vi "Start DAQ.vi"(8 "error in (no error)":errorcluster, 10 "Run info in":T1, 11 "Sampling info in":T2={"Channels"=[], "Sampling freq"=0, "Output freq"=0, "Update freq"=0, "Steps per rev"=0, "Counts per rev"=0, "Amplifier"="", "Motor driver"="", "Step bit"=0, "Max speed"=0.0, "Max accel"=0.0, "Pos gain"=0.0, "Vel gain"=0.0, "counter"="Dev1/ctr0"} {"Channels"."Hi cutoff" items=["500"=500.0, "1k"=1000.0, "5k"=5000.0, "10k"=10000.0, "20k"=20000.0]; "Channels"."Lo cutoff" items=["0.1"=0.1, "1"=1.0, "10"=10.0, "100"=100.0, "300"=300.0]; "Channels"."Gain" items=["x100"=100, "x1000"=1000, "x10000"=10000]}) -> (0 "error out":errorcluster, 1 "start time":timestamp, 2 "Run info":T1, 3 "Sampling info out":T2={"Channels"=[], "Sampling freq"=0, "Output freq"=0, "Update freq"=0, "Steps per rev"=0, "Counts per rev"=0, "Amplifier"="", "Motor driver"="", "Step bit"=0, "Max speed"=0.0, "Max accel"=0.0, "Pos gain"=0.0, "Vel gain"=0.0, "counter"="Dev1/ctr0"} {"Channels"."Hi cutoff" items=["500"=500.0, "1k"=1000.0, "5k"=5000.0, "10k"=10000.0, "20k"=20000.0]; "Channels"."Lo cutoff" items=["0.1"=0.1, "1"=1.0, "10"=10.0, "100"=100.0, "300"=300.0]; "Channels"."Gain" items=["x100"=100, "x1000"=1000, "x10000"=10000]})   [LabVIEW 2012]
uses:
  Sampling info.ctl
  Channel.ctl
  Run info.ctl
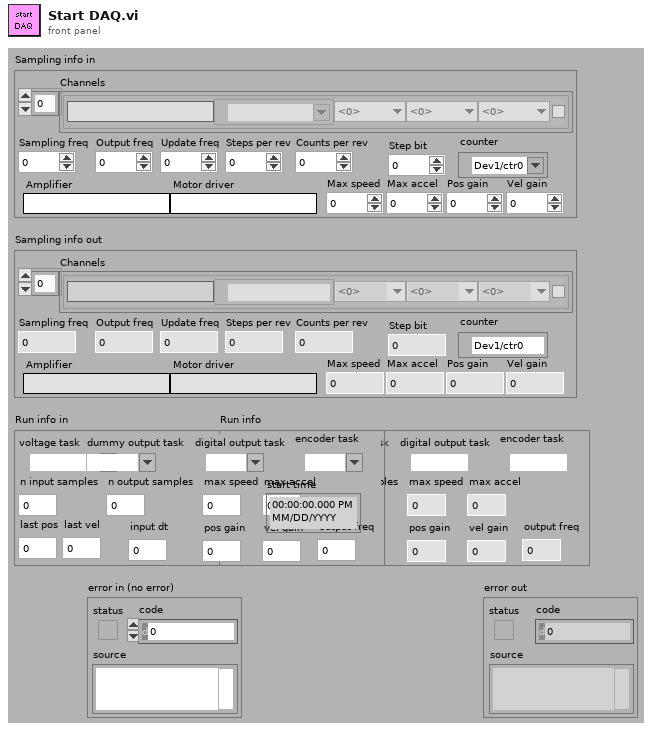
[diagram p1: front panel]
types:
  T1 = typedef "Run info.ctl" = cluster{"voltage task":refnum<k21>, "dummy output task":refnum<k21>, "digital output task":refnum<k21>, "encoder task":refnum<k21>, "n input samples":i32, "n output samples":i32, "max speed":dbl, "max accel":dbl, "last pos":dbl, "last vel":dbl, "pos gain":dbl, "vel gain":dbl, "input dt":dbl, "output freq":dbl}
  T2 = typedef "Sampling info.ctl" = cluster{"Channels":T3[], "Sampling freq":i32, "Output freq":i32, "Update freq":i32, "Steps per rev":i32, "Counts per rev":i32, "Amplifier":string, "Motor driver":string, "Step bit":u8, "Max speed":dbl, "Max accel":dbl, "Pos gain":dbl, "Vel gain":dbl, "counter":tag}
  T3 = typedef "Channel.ctl" = cluster{"Name":string, "Chan":tag, "Gain":u16, "Lo cutoff":dbl, "Hi cutoff":dbl, "Notch":bool}
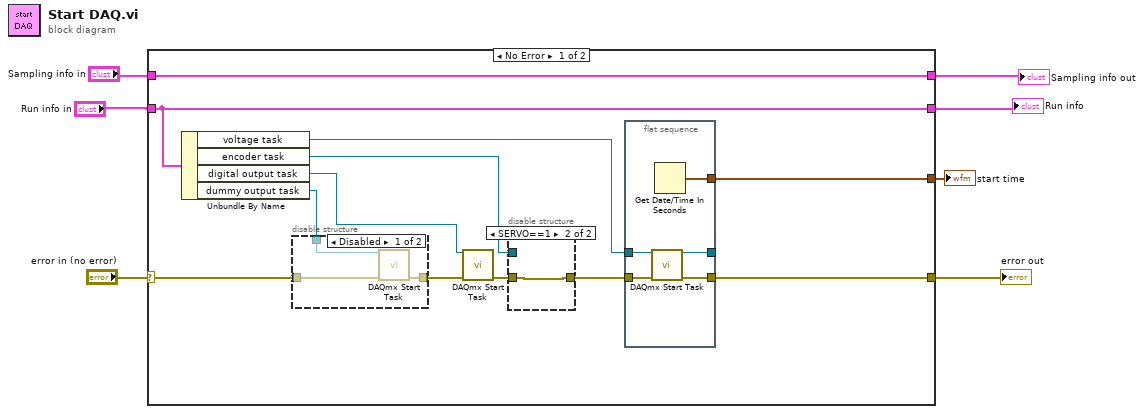
[diagram p0: block diagram]
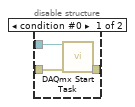
[diagram p2: hidden frame]
diagram:
  n1 = case shown="No Error" "error in (no error)" {
    selector: "error in (no error)" -> [w17 w34]
    tunnel: [w12 w33] -> w3
    tunnel: [w14 w34] -> w6
    tunnel: [w19 w35] -> w2
    tunnel: "Sampling info in" -> [w19 w35]
    tunnel: "Run info in" -> [w12 w33]
    tunnel: [w13 _] -> w1
    frame No Error {
      n2 = Unbundle By Name(w12) -> ("voltage task"=w15:refnum<k21>, "encoder task"=w10:refnum<k21>, "digital output task"=w16:refnum<k21>, "dummy output task"=w18:refnum<k21>)
      n3 = disable-structure shown="Disabled" {
        disable-tunnel: w18 -> [w26 _]
        disable-tunnel: w17 -> [w25 w27]
        disable-tunnel: [w24 w27] -> w11
        frame Disabled {
          n4 = call <vilib>:"DAQmx Start Task.vi"("task/channels in"=w26, "error in"=w25) -> ("error out"=w24:errorcluster)  [unwired: 12 in, 1 out]
        }
        frame Enabled {
        }
      }
      n5 = call <vilib>:"DAQmx Start Task.vi"("task/channels in"=w16, "error in"=w11) -> ("error out"=w9:errorcluster)  [unwired: 12 in, 1 out]
      n6 = disable-structure shown="SERVO==1" {
        disable-tunnel: w10 -> [w22 _]
        disable-tunnel: w9 -> [w21 w23]
        disable-tunnel: [w20 w23] -> w8
        frame condition #0 {
          n7 = call <vilib>:"DAQmx Start Task.vi"("task/channels in"=w22, "error in"=w21) -> ("error out"=w20:errorcluster)  [unwired: 12 in, 1 out]
        }
        frame condition #1 (active) {
        }
      }
      n8 = flat-sequence {
        tunnel: w8 -> [w32]
        tunnel: w15 -> [w31]
        tunnel: [w30] -> w13
        tunnel: [w29] -> _
        tunnel: [w28] -> w14
        frame #0 {
          n9 = call <vilib>:"DAQmx Start Task.vi"("task/channels in"=w31, "error in"=w32) -> ("task out"=w29:refnum<k21>, "error out"=w28:errorcluster)  [unwired: 12 in]
          n10 = Get Date/Time In Seconds() -> (seconds since 1Jan1904=w30:timestamp)
        }
      }
    }
    frame Error {
    }
  }
  "error out" <- w6
  "Run info" <- w3
  "Sampling info out" <- w2
  "start time" <- w1
